vi "Banana_Greater Value Comparison.vi"(6 "verbose? (F)":bool, 8 "error in (no error)":errorcluster, 9 "Y":variant, 10 "X":variant, 11 "Less Than? (F)":bool) -> (0 "error out":errorcluster, 2 "Asserted?":bool, 3 "Verbose output":string)   [LabVIEW 2021, in "Bananas.lvlib"]
uses:
  Bananas.lvlib
  <vilib>/Utility/VariantDataType/Type.ctl
  <vilib>/Utility/VariantDataType/VariantType.lvlib
  <vilib>/Utility/Data Type/NI_Data Type.lvlib
  <vilib>/LabVIEW Open Source Project/Data Manipulation/Variant/OpenVariant.lvlib
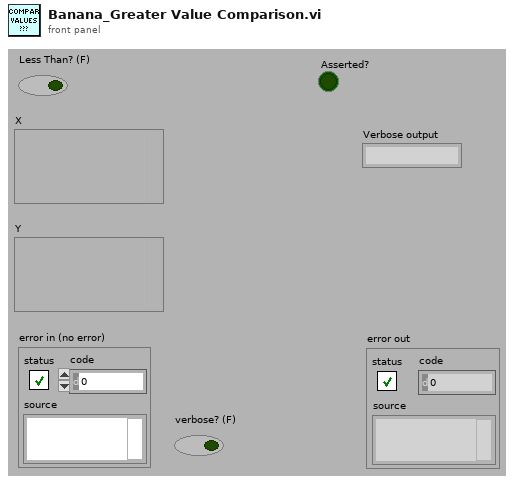
[diagram p1: front panel]
types:
  T1 = typedef "VariantType.lvlib/Type.ctl" = enum8{"Invalid Type", "Void", "I8", "I16", "I32", "I64", "U8", "U16", "U32", "U64", "Single Float", "Double Float", "Extended Float", "Single Complex", "Double Complex", "Extended Complex", "Enum U8", "Enum U16", "Enum U32", "Enum U64", "Single Float With Unit", "Double Float With Unit", "Extended Float With Unit", "Single Complex with Unit", "Double Complex with Unit", "Extended Complex with Unit", "Boolean", "String", "Path", "Picture", "Tag", "Array", "Cluster", "Variant", "LV Variant", "Waveform", "Timestamp", "Digital Waveform", "Digital Data", "ExpressData", "Refnum", "External Data", "VI", "Poly VI", "LabVIEW Class Instance", "Fixed Point"}
  T2 = typedef "NI_Data Type.lvlib/Data Type.ctl" = enum8{"Invalid Type", "Void", "I8", "I16", "I32", "I64", "U8", "U16", "U32", "U64", "Single Float", "Double Float", "Extended Float", "Single Complex", "Double Complex", "Extended Complex", "Enum U8", "Enum U16", "Enum U32", "Enum U64", "Single Float With Unit", "Double Float With Unit", "Extended Float With Unit", "Single Complex with Unit", "Double Complex with Unit", "Extended Complex with Unit", "Boolean", "String", "Path", "Picture", "Tag", "Array", "Cluster", "Variant", "LV Variant", "Waveform", "Timestamp", "Digital Waveform", "Digital Data", "ExpressData", "Refnum", "External Data", "VI", "Poly VI", "LabVIEW Class Instance", "Fixed Point", "Set Collection", "Map Collection"}
  T3 = typedef "NI_Data Type.lvlib/Unit Info.ctl" = cluster{"Unit Type":T4, "Exponent":i16}
  T4 = typedef "NI_Data Type.lvlib/Unit Type.ctl" = enum16{"Radians", "Steradians", "Seconds", "Meters", "Kilograms", "Amperes", "Kelvins", "Moles", "Candelas", "InvalidUnit"}
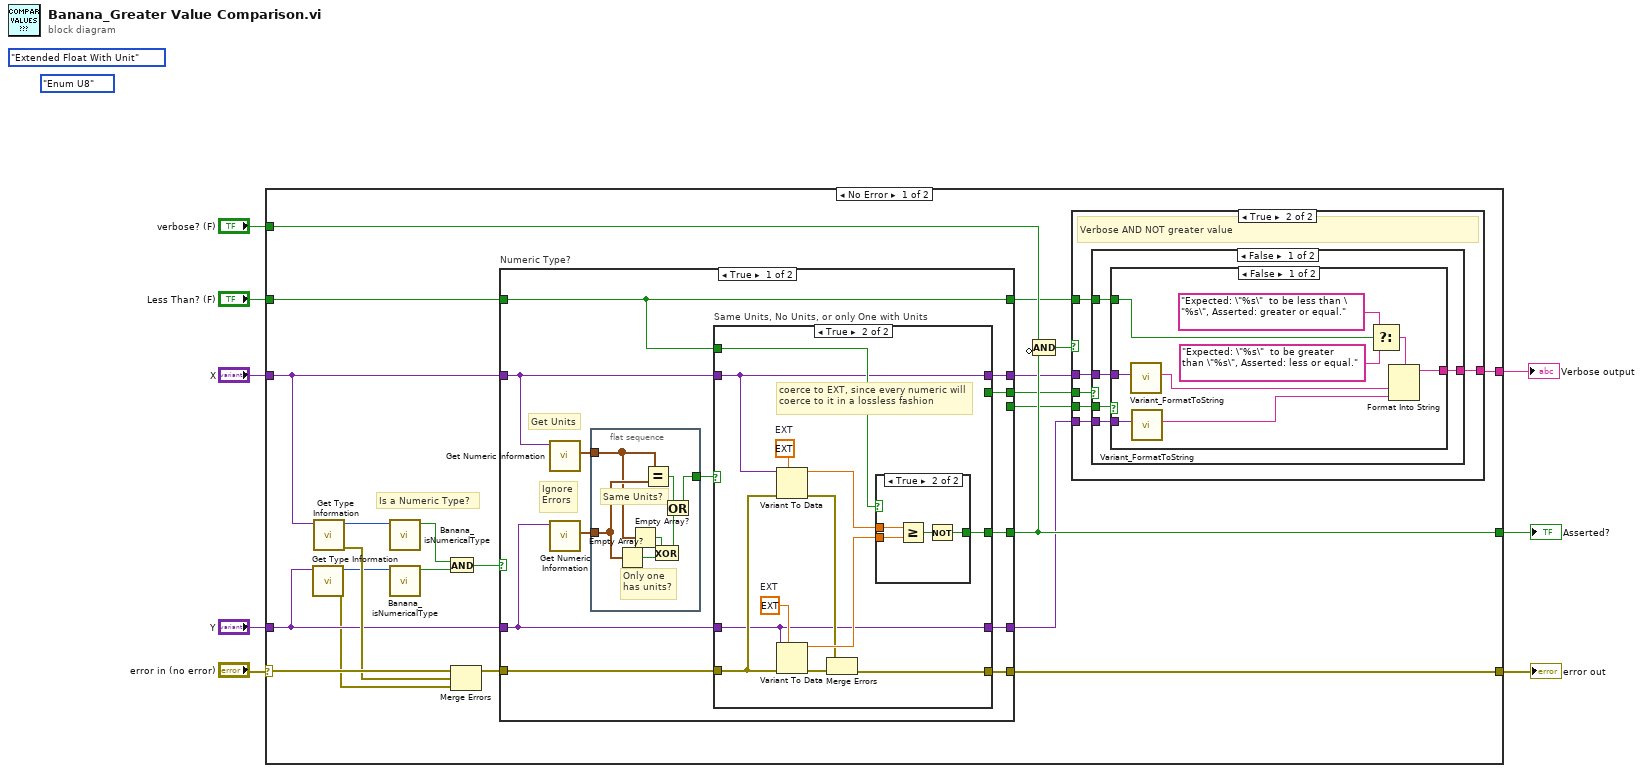
[diagram p0: block diagram]
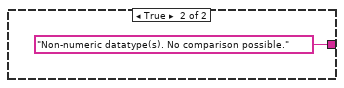
[diagram p3: hidden frame]
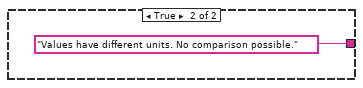
[diagram p4: hidden frame]
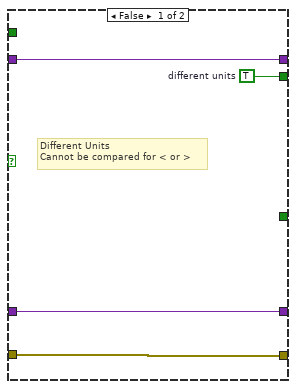
[diagram p5: hidden frame]
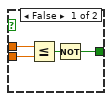
[diagram p6: hidden frame]
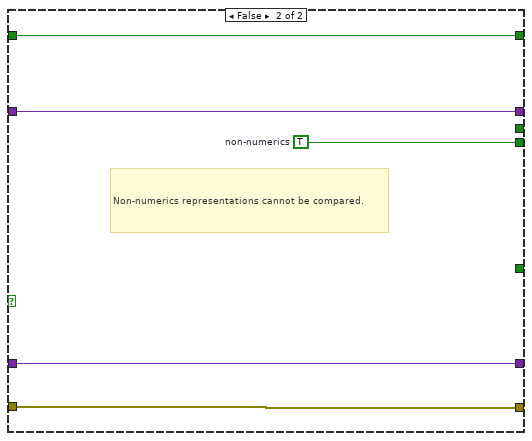
[diagram p7: hidden frame]
diagram:
  (unwired) Type."Enum U8" ("Type Enum")
  (unwired) Type."Extended Float With Unit" ("Type Enum")
  n1 = case shown="No Error" "error in (no error)" {
    selector: "error in (no error)" -> [w19 w101]
    tunnel: [w30 _] -> w8
    tunnel: [w29 w101] -> w7
    tunnel: "Y" -> [w11 _]
    tunnel: "verbose? (F)" -> [w27 _]
    tunnel: [w26 _] -> w4
    tunnel: "Less Than? (F)" -> [w25 _]
    tunnel: "X" -> [w14 _]
    frame No Error {
      # "Is a Numeric Type?"
      n2 = call <vilib>:"Get Type Information.vi"("variant"=w11) -> ("error out"=w9:errorcluster, "type"=w10:T2)  [unwired: 6 in, 3 out]
      n3 = call <vilib>:"Get Type Information.vi"("variant"=w14) -> ("error out"=w12:errorcluster, "type"=w13:T2)  [unwired: 6 in, 3 out]
      n4 = call "Banana_isNumericalType.vi"("Type Enum"=w13) -> ("is Numeric"=w16:bool)  [unwired: 10 in]
      n5 = call "Banana_isNumericalType.vi"("Type Enum"=w10) -> ("is Numeric"=w15:bool)  [unwired: 10 in]
      n6 = And(x=w16, y=w15) -> (x .and. y?=w20:bool)
      n7 = Merge Errors(w19, w12, w9) -> (w28:errorcluster)
      n8 = case "Numeric Type?" shown="True" w20 {
        tunnel: w14 -> [w53 w96]
        tunnel: w11 -> [w56 w97]
        tunnel: [w64 _] -> w30
        tunnel: w28 -> [w62 w100]
        tunnel: [w63 w100] -> w29
        tunnel: [w60 _] -> w23
        tunnel: [_ w99] -> w22
        tunnel: w25 -> [w59 w98]
        tunnel: [w59 w98] -> w21
        tunnel: [w57 w97] -> w18
        tunnel: [w58 w96] -> w17
        frame True {
          # "Get Units"
          # "Ignore\nErrors"
          n9 = call <vilib>:"Get Numeric Information.vi"("variant"=w53) -> ("units"=w54:T3[])  [unwired: 7 in, 3 out]
          n10 = call <vilib>:"Get Numeric Information.vi"("variant"=w56) -> ("units"=w55:T3[])  [unwired: 7 in, 3 out]
          n11 = flat-sequence {
            tunnel: w54 -> [w94]
            tunnel: w55 -> [w95]
            tunnel: [w89] -> w61
            frame #0 {
              # "Same Units?"
              # "Only one\nhas units?"
              n12 = Empty Array?(array=w95) -> (empty?=w93:bool)
              n13 = Empty Array?(array=w94) -> (empty?=w92:bool)
              n14 = Equal?(x=w94, y=w95) -> (x = y?=w90:bool)
              n15 = Exclusive Or(1:w93, 2:w92) -> (0:w91:bool)
              n16 = Or(x=w90, y=w91) -> (x .or. y?=w89:bool)
            }
          }
          n17 = case "Same Units, No Units, or only One with Units" shown="True" w61 {
            tunnel: [_ w80] -> w64
            tunnel: [w68 w74] -> w63
            tunnel: w53 -> [w66 w70]
            tunnel: w56 -> [w65 w69]
            tunnel: w62 -> [w68 w76]
            tunnel: [w67 _] -> w60
            tunnel: w59 -> [_ w73]
            tunnel: [w66 w70] -> w58
            tunnel: [w65 w69] -> w57
            frame False {
              w67 = TRUE  # different units
              # "Different Units\nCannot be compared for < or >"
            }
            frame True {
              w71 = ext 0.0  # EXT
              w72 = ext 0.0  # EXT
              # "coerce to EXT, since every numeric will coerce to it in a lossless fashion"
              n18 = Variant To Data(error in=w76, type=w72, Variant=w70) -> (data=w78:ext, error out=w77:errorcluster)
              n19 = Variant To Data(error in=w76, type=w71, Variant=w69) -> (data=w79:ext, error out=w75:errorcluster)
              n20 = Merge Errors(w77, w75) -> (w74:errorcluster)
              n21 = case shown="True" w73 {
                tunnel: [w81 w85] -> w80
                tunnel: w79 -> [w84 w87]
                tunnel: w78 -> [w83 w86]
                frame False {
                  n22 = Less Or Equal?(x=w83, y=w84) -> (x <= y?=w82:bool)
                  n23 = Not(x=w82) -> (.not. x?=w81:bool)
                }
                frame True {
                  n24 = Greater Or Equal?(x=w86, y=w87) -> (x >= y?=w88:bool)
                  n25 = Not(x=w88) -> (.not. x?=w85:bool)
                }
              }
            }
          }
        }
        frame False {
          w99 = TRUE  # non-numerics
          # "Non-numerics representations cannot be compared."
        }
      }
      n26 = Compound Arithmetic op=AND(w27, invert w30) -> (w24:bool)
      n27 = case shown="True" w24 {
        tunnel: [_ w36] -> w26
        tunnel: w17 -> [_ w35]
        tunnel: w18 -> [_ w34]
        tunnel: w23 -> [_ w33]
        tunnel: w22 -> [_ w32]
        tunnel: w21 -> [_ w31]
        frame False {
        }
        frame True {
          # "Verbose AND NOT greater value"
          n28 = case shown="False" w33 {
            tunnel: [w41 "Values have different units. No comparison possible." ("format string")] -> w36
            tunnel: w35 -> [w40 _]
            tunnel: w34 -> [w39 _]
            tunnel: w32 -> [w38 _]
            tunnel: w31 -> [w37 _]
            frame False {
              n29 = case shown="False" w38 {
                tunnel: [w50 "Non-numeric datatype(s). No comparison possible." ("format string")] -> w41
                tunnel: w40 -> [w42 _]
                tunnel: w39 -> [w45 _]
                tunnel: w37 -> [w49 _]
                frame False {
                  n30 = call <vilib>:"Variant_FormatToString.vi"("Variant"=w42) -> ("Value"=w43:string)  [unwired: 10 in]
                  n31 = call <vilib>:"Variant_FormatToString.vi"("Variant"=w45) -> ("Value"=w44:string)  [unwired: 10 in]
                  n32 = Select(t="Expected: \"%s\"  to be less than \"%s\", Asserted: greater or equal.", s=w49, f="Expected: \"%s\"  to be greater than \"%s\", Asserted: less or equal." ("t")) -> (s? t:f=w48:string)
                  n33 = Format Into String(format string=w48, w43, w44) -> (resulting string=w50:string)  [unwired: 2 in, 1 out]
                }
                frame True {
                }
              }
            }
            frame True {
            }
          }
        }
      }
    }
    frame Error {
    }
  }
  "Asserted?" <- w8
  "error out" <- w7
  "Verbose output" <- w4
